vi "JWSH-515S-W1D.vi"(7 "地址":string="01", 8 "TestIndex":i32) -> (0 "humidity":dbl format="%.1f", 2 "temperature":dbl format="%.1f", 3 "result":bool)   [LabVIEW 2015]
uses:
  <vilib>/Instr/_visa.llb/VISA Configure Serial Port (Instr).vi
panel:
  out "AC电源":refnum<visa-resource-name>
  out "读取缓冲区":string
  out "字符串":string
  out "错误输出":errorcluster
  # "温湿度输出"
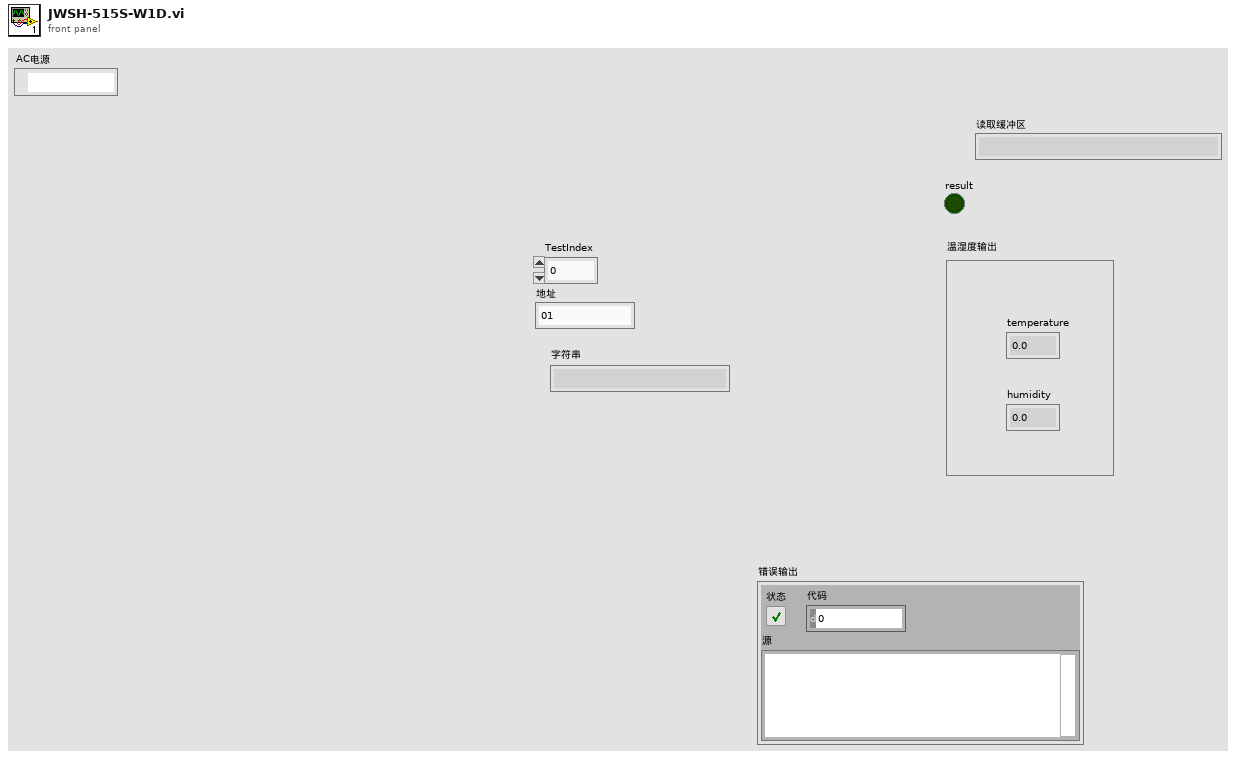
[diagram p1: front panel]
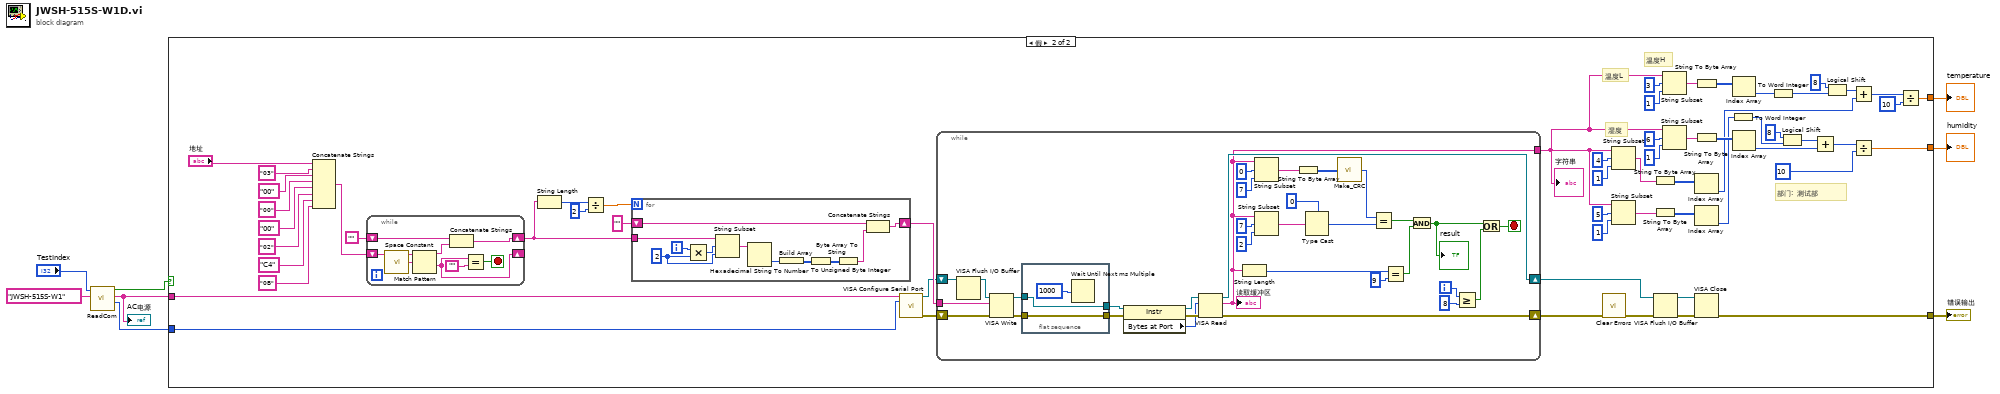
[diagram p0: block diagram]
diagram:
  n1 = call "ReadCom.vi"("仪器名称"="JWSH-515S-W1", "MyIndex"="TestIndex") -> ("Baudrate"=w2:i32, "COM"=w3:string, "OK?"=w6:bool)  [unwired: 7 in]
  "AC电源" <- w3
  n2 = case shown="假" w6 {
    tunnel: [_ w65] -> w8
    tunnel: [_ w64] -> w7
    tunnel: w3 -> [_ w63]
    tunnel: w2 -> [_ w62]
    tunnel: [_ w10] -> w1
    frame True {
    }
    frame False {
      # "部门:  测试部"
      # "温度L"
      # "湿度"
      # "温度H"
      n3 = Concatenate Strings("地址", "03", "00", "00", "00", "02", "C4", "0B") -> (w60:string)
      n4 = while {
        shift-right: [w120] -> _
        shift-left: w60 -> [w115]
        shift-right: [w116] -> w67
        shift-left: "" -> [w118]
        stop <- w119 stop-if-true
        n5 = call <vilib>:"Space Constant.vi"() -> ("String"=w122:string)
        n6 = Match Pattern(string=w115, regular expression=w122) -> (before substring=w117:string, after substring=w120:string)  [unwired: 1 in, 2 out]
        n7 = Concatenate Strings(w118, w117) -> (w116:string)
        n8 = Equal?(x=w120, y="") -> (x = y?=w119:bool)
      }
      n9 = String Length(string=w67) -> (length=w50:i32)
      n10 = Divide(x=w50, y=2) -> (x/y=w52:dbl)
      n11 = for {
        N: w52 -> [_]
        shift-right: [w114] -> w48
        shift-left: "" -> [w113]
        tunnel: w67 -> [w109]
        i -> [w108]
        w106 = 2
        n12 = Multiply(x=w108, y=w106) -> (x*y=w107:i32)
        n13 = String Subset(string=w109, offset (0)=w107, length (rest)=w106) -> (substring=w110:string)
        n14 = Hexadecimal String To Number(string=w110) -> (number=w111:u32)  [unwired: 2 in, 1 out]
        n15 = Build Array(w111) -> (w105:u32[])
        n16 = To Unsigned Byte Integer(number=w105) -> (unsigned 8bit integer=w104:u8[])
        n17 = Byte Array To String(unsigned byte array=w104) -> (string=w112:string)
        n18 = Concatenate Strings(w113, w112) -> (w114:string)
      }
      n19 = call-poly "VISA Configure Serial Port"("VISA resource name"=w63, "baud rate (9600)"=w62) -> ("VISA resource name out"=w42:refnum<visa-resource-name>, "error out"=w41:errorcluster)  [unwired: 12 in]
      n20 = while {
        tunnel: w48 -> [w99]
        tunnel: [w75] -> w66
        shift-right: [w93] -> w47
        shift-left: w41 -> [w100]
        shift-right: [w92] -> w45
        shift-left: w42 -> [w69]
        i -> [w79]
        stop <- w76 stop-if-true
        n21 = VISA Flush I/O Buffer(VISA resource name=w69) -> (VISA resource name out=w68:refnum<visa-resource-name>)  [unwired: 2 in, 1 out]
        n22 = VISA Write(VISA resource name=w68, write buffer=w99, error in (no error)=w100) -> (VISA resource name out=w98:refnum<visa-resource-name>, error out=w90:errorcluster)  [unwired: 1 out]
        n23 = flat-sequence {
          tunnel: [w102] -> w97
          tunnel: w98 -> [w102]
          tunnel: w90 -> [w101]
          tunnel: [w101] -> w91
          frame #0 {
            n24 = Wait Until Next ms Multiple(millisecond multiple=u32 1000 ("毫秒倍数")) -> ()  [unwired: 1 out]
          }
        }
        n25 = property class="Instr"(reference=w97, error in=w91) -> (reference out=w96:refnum<visa-resource-name>, error out=w95:errorcluster, "Bytes at Port"=w94:u32)
        n26 = VISA Read(VISA resource name=w96, byte count=w94, error in (no error)=w95) -> (VISA resource name out=w92:refnum<visa-resource-name>, read buffer=w75:string, error out=w93:errorcluster)  [unwired: 1 out]
        "读取缓冲区" <- w75
        n27 = String Length(string=w75) -> (length=w74:i32)
        n28 = String Subset(string=w75, offset (0)=0, length (rest)=7) -> (substring=w82:string)
        n29 = String Subset(string=w75, offset (0)=7, length (rest)=2) -> (substring=w88:string)
        n30 = String To Byte Array(string=w82) -> (unsigned byte array=w85:u8[])
        n31 = Type Cast(type=u16 0, x=w88) -> (*(type *) &x=w80:u16)
        n32 = call "Make_CRC.vi"("数组输入"=w85) -> ("CRC_反"=w81:u16)
        n33 = Equal?(x=w81, y=w80) -> (x = y?=w71:bool)
        n34 = Equal?(x=w74, y=9) -> (x = y?=w72:bool)
        n35 = And(x=w71, y=w72) -> (x .and. y?=w70:bool)
        "result" <- w70
        n36 = Greater Or Equal?(x=w79, y=8) -> (x >= y?=w77:bool)
        n37 = Or(x=w70, y=w77) -> (x .or. y?=w76:bool)
      }
      "字符串" <- w66
      n38 = call <vilib>:"Clear Errors.vi"("error in (no error)"=w47) -> ("error out"=w46:errorcluster)  [unwired: 5 in, 1 out]
      n39 = String Subset(string=w66, offset (0)=4, length (rest)=1 ("长度（剩余）")) -> (substring=w30:string)
      n40 = String Subset(string=w66, offset (0)=5, length (rest)=1) -> (substring=w23:string)
      n41 = String To Byte Array(string=w30) -> (unsigned byte array=w29:u8[])
      n42 = String To Byte Array(string=w23) -> (unsigned byte array=w22:u8[])
      n43 = VISA Flush I/O Buffer(VISA resource name=w45, error in (no error)=w46) -> (VISA resource name out=w43:refnum<visa-resource-name>, error out=w44:errorcluster)  [unwired: 1 in]
      n44 = String Subset(string=w66, offset (0)=3, length (rest)=1 ("长度（剩余）")) -> (substring=w34:string)
      n45 = String Subset(string=w66, offset (0)=6, length (rest)=1) -> (substring=w37:string)
      n46 = String To Byte Array(string=w34) -> (unsigned byte array=w36:u8[])
      n47 = String To Byte Array(string=w37) -> (unsigned byte array=w35:u8[])
      n48 = Index Array(array=w29) -> (element=w26:u8)  [unwired: 1 in]
      n49 = Index Array(array=w22) -> (element=w12:u8)  [unwired: 1 in]
      n50 = VISA Close(VISA resource name=w43, error in (no error)=w44) -> (error out=w10:errorcluster)
      n51 = To Word Integer(number=w12) -> (16bit integer=w11:i16)
      n52 = Index Array(array=w36) -> (element=w14:u8)  [unwired: 1 in]
      n53 = Index Array(array=w35) -> (element=w19:u8)  [unwired: 1 in]
      n54 = To Word Integer(number=w14) -> (16bit integer=w13:i16)
      n55 = Logical Shift(y=8, x=w11) -> (x << y=w20:i16)
      n56 = Add(x=w20, y=w19) -> (x+y=w15:i16)
      n57 = Logical Shift(y=8, x=w13) -> (x << y=w27:i16)
      n58 = Add(x=w27, y=w26) -> (x+y=w16:i16)
      n59 = Divide(x=w15, y=10) -> (x/y=w64:dbl)
      n60 = Divide(x=w16, y=10) -> (x/y=w65:dbl)
    }
  }
  "temperature" <- w8
  "humidity" <- w7
  "错误输出" <- w1
